vi "CloneAndConditionReferenceWaveform.vi"(0 "Reference Waveform":T1 {"Runtime Scaling" format="%#_6p"; "Sample Rate" format="%#_6p"; "Burst Length (s)" format="%#_6p"; "PAPR (dB)" format="%.2f"; "Signal Bandwidth (Hz)" format="%#_6p"}, 11 "error in (no error)":errorcluster) -> (4 "Conditioned Reference Waveform":T1 {"Runtime Scaling" format="%#_6p"; "Sample Rate" format="%#_6p"; "Burst Length (s)" format="%#_6p"; "PAPR (dB)" format="%.2f"; "Signal Bandwidth (Hz)" format="%#_6p"}, 15 "error out":errorcluster)   [LabVIEW 2016, in "Envelope Tracking.lvlib"]
uses:
  Envelope Tracking.lvlib
  Common/Waveform.ctl
  Common/Common.lvlib
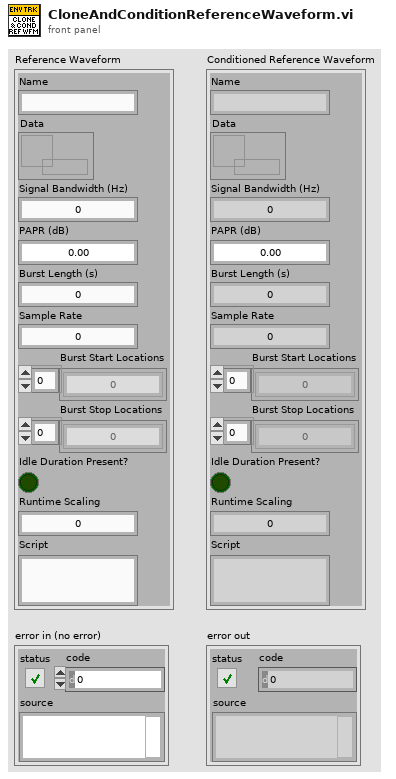
[diagram p1: front panel]
types:
  T1 = typedef "Common.lvlib/Waveform.ctl" = cluster{"Name":string, "Data":refnum<data-value>, "Signal Bandwidth (Hz)":dbl, "PAPR (dB)":dbl, "Burst Length (s)":dbl, "Sample Rate":dbl, "Burst Start Locations":i32[], "Burst Stop Locations":i32[], "Idle Duration Present?":bool, "Runtime Scaling":dbl, "Script":string}
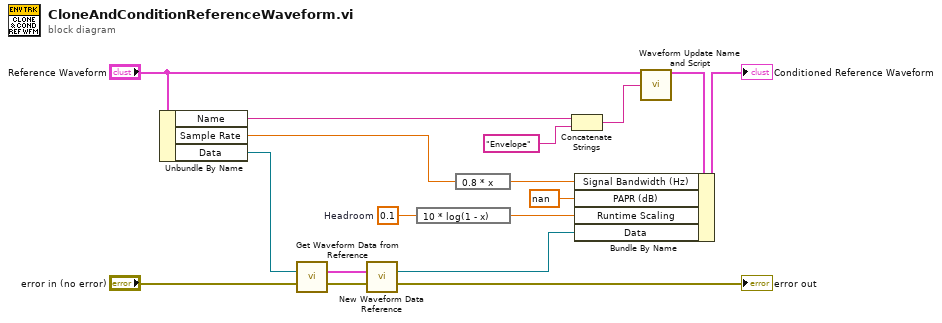
[diagram p0: block diagram]
diagram:
  w9 = 0.1  # Headroom
  n1 = Unbundle By Name("Reference Waveform") -> ("Name"=w16:string, "Sample Rate"=w12:dbl, "Data"=w6:refnum<data-value>)
  n2 = call "Get Waveform Data from Reference.vi"("Waveform Data Reference"=w6, "error in (no error)"="error in (no error)") -> ("Waveform Data"=w5:cluster{"t0":dbl, "dt":dbl, "y":csg[]}, "error out"=w4:errorcluster)  [unwired: 12 in]
  n3 = call "New Waveform Data Reference.vi"("Waveform Data"=w5, "error in (no error)"=w4) -> ("Waveform Data Reference"=w3:refnum<data-value>, "error out"=→"error out":errorcluster)  [unwired: 12 in]
  n4 = expression code="10 * log(1 - x)"(w9) -> (w8:dbl)
  n5 = expression code="0.8 * x"(w12) -> (w11:dbl)
  n6 = Concatenate Strings(w16, "Envelope" ("string")) -> (w14:string)
  n7 = call "Waveform Update Name and Script.vi"("Waveform in"="Reference Waveform", "New Waveform Name"=w14) -> ("Waveform out"=w13:T1)  [unwired: 13 in]
  n8 = Bundle By Name(cluster=w13, "Signal Bandwidth (Hz)"=w11, "PAPR (dB)"=nan, "Runtime Scaling"=w8, "Data"=w3) -> (→"Conditioned Reference Waveform":T1)
